vi "Dashboard Cell Resize.vi"(6 "Cluster":T1={"Label Font Size"=24, "Data Font Size"=36, "String Font Size"=36}, 8 "error in (no error)":errorcluster, 9 "Cluster Size:Height":u32=134, 10 "Cluster Size:Width":u32=256, 11 "引气压力P4 4":refnum<vi>) -> (0 "error out":errorcluster, 1 "Bounds:Area Height":u32=134, 2 "Bounds:Area Width":u32=256)   [LabVIEW 2014, in "jkism-tool-support.lvlib"]
uses:
  jkism-tool-support.lvlib
panel:
  out "引气压力P4 2":T2={"Label"="Label", "Value"="0.00", "String"="0.00"} caption="Digital"
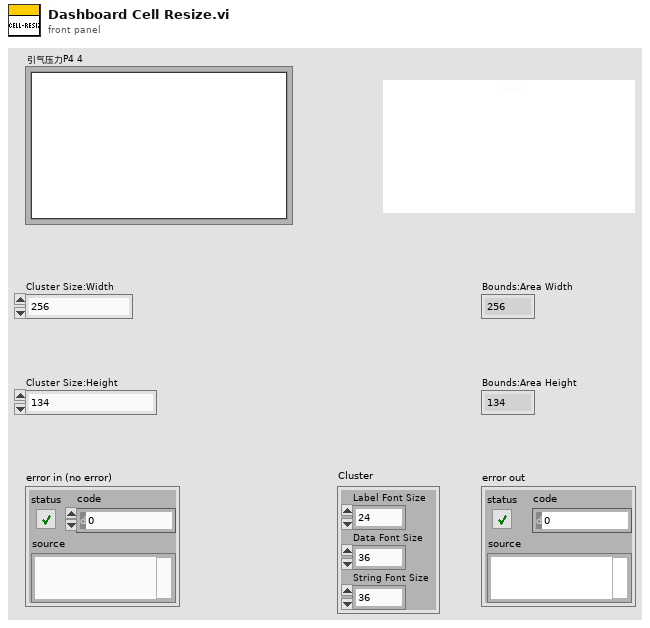
[diagram p1: front panel]
types:
  T1 = cluster{"Label Font Size":i32, "Data Font Size":i32, "String Font Size":i32}
  T2 = cluster{"Label":string, "Value":string, "String":string}
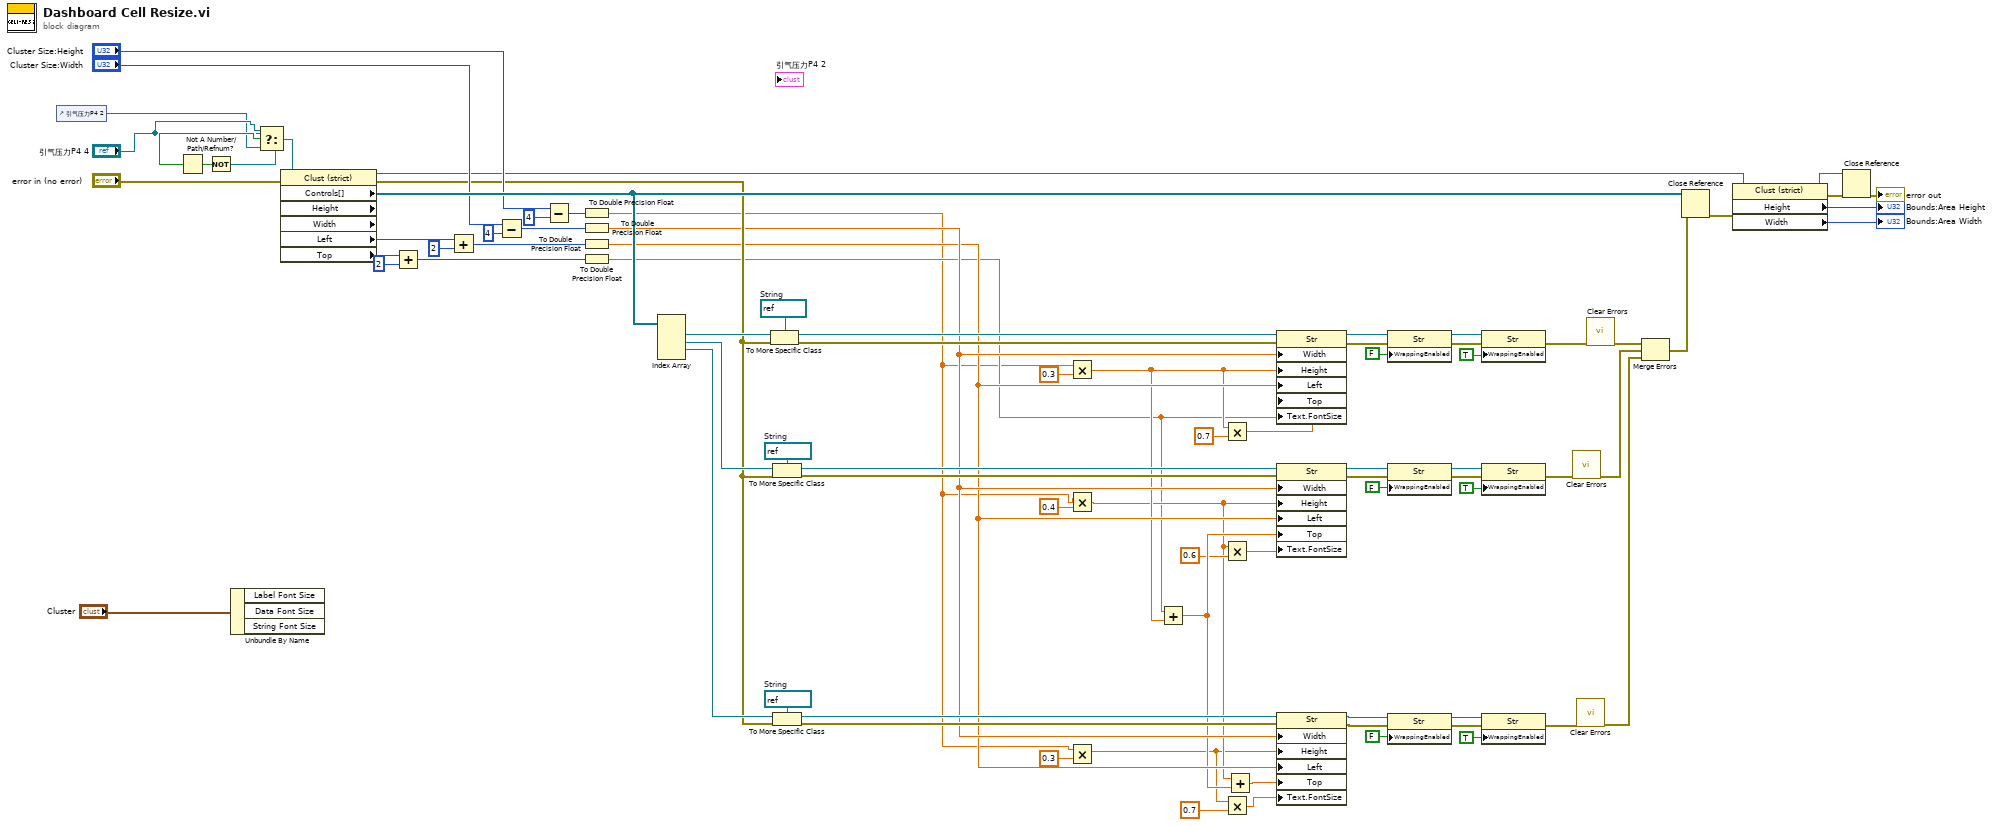
[diagram p0: block diagram]
diagram:
  w47 = refnum<vi> refnum  # String
  w78 = refnum<vi> refnum  # String
  w82 = refnum<vi> refnum  # String
  n1 = control-ref of="引气压力P4 2"() -> (w53:refnum<vi>)
  n2 = Not A Number/Path/Refnum?(number/path/refnum="引气压力P4 4") -> (NaN/Path/Refnum?=w1:bool)
  n3 = Not(x=w1) -> (.not. x?=w55:bool)
  n4 = Unbundle By Name("Cluster") -> ()  [unwired: 3 out]
  n5 = Select(t="引气压力P4 4", s=w55, f=w53) -> (s? t:f=w52:refnum<vi>)
  n6 = property on="Property Node" class="Clust (strict)" props=["Controls[]", "Height", "Width", "Left", "Top"](reference=w52, error in="error in (no error)") -> (reference out=w59:refnum<vi>, error out=w44:errorcluster, "Controls[]"=w83:refnum<vi>[], "Left"=w72:i32, "Top"=w69:i32)  [unwired: 2 out]
  n7 = Add(x=w69, y=2) -> (x+y=w50:i32)
  n8 = Add(x=w72, y=2) -> (x+y=w68:i32)
  n9 = Subtract(x="Cluster Size:Width", y=u32 4) -> (x-y=w75:u32)
  n10 = Subtract(x="Cluster Size:Height", y=u32 4) -> (x-y=w51:u32)
  n11 = To Double Precision Float(number=w51) -> (double precision float=w26:dbl)
  n12 = To Double Precision Float(number=w75) -> (double precision float=w43:dbl)
  n13 = To Double Precision Float(number=w68) -> (double precision float=w42:dbl)
  n14 = To Double Precision Float(number=w50) -> (double precision float=w30:dbl)
  n15 = Index Array(array=w83) -> (element #1=w80:refnum<vi>, element #2=w77:refnum<vi>, element #3=w45:refnum<vi>)  [unwired: 4 in, 1 out]
  n16 = To More Specific Class(target class=w82, reference=w80, error in=w44) -> (specific class reference=w81:refnum<vi>, error out=w65:errorcluster)
  n17 = To More Specific Class(target class=w78, reference=w77, error in=w44) -> (specific class reference=w79:refnum<vi>, error out=w66:errorcluster)
  n18 = To More Specific Class(target class=w47, reference=w45, error in=w44) -> (specific class reference=w46:refnum<vi>, error out=w48:errorcluster)
  n19 = Multiply(x=w26, y=0.3) -> (x*y=w37:dbl)
  n20 = Multiply(x=w26, y=0.4) -> (x*y=w32:dbl)
  n21 = Multiply(x=w26, y=0.3) -> (x*y=w28:dbl)
  n22 = Add(x=w30, y=w37) -> (x+y=w41:dbl)
  n23 = Multiply(x=w37, y=0.7) -> (x*y=w38:dbl)
  n24 = Multiply(x=w32, y=0.6) -> (x*y=w33:dbl)
  n25 = Multiply(x=w28, y=0.7) -> (x*y=w29:dbl)
  n26 = Add(x=w32, y=w41) -> (x+y=w49:dbl)
  n27 = property on="Property Node" class="Str"(reference=w81, error in=w65, "Width"=w43, "Height"=w37, "Left"=w42, "Top"=w30, "Text.FontSize"=w38) -> (reference out=w22:refnum<vi>, error out=w21:errorcluster)
  n28 = property on="Property Node" class="Str"(reference=w79, error in=w66, "Width"=w43, "Height"=w32, "Left"=w42, "Top"=w41, "Text.FontSize"=w33) -> (reference out=w10:refnum<vi>, error out=w11:errorcluster)
  n29 = property on="Property Node" class="Str"(reference=w46, error in=w48, "Width"=w43, "Height"=w28, "Left"=w42, "Top"=w49, "Text.FontSize"=w29) -> (reference out=w4:refnum<vi>, error out=w3:errorcluster)
  n30 = property on="Property Node" class="Str"(reference=w22, error in=w21, "WrappingEnabled"=FALSE ("Enable Wrapping")) -> (reference out=w17:refnum<vi>, error out=w18:errorcluster)
  n31 = property on="Property Node" class="Str"(reference=w10, error in=w11, "WrappingEnabled"=FALSE ("Enable Wrapping")) -> (reference out=w15:refnum<vi>, error out=w14:errorcluster)
  n32 = property on="Property Node" class="Str"(reference=w4, error in=w3, "WrappingEnabled"=FALSE ("Enable Wrapping")) -> (reference out=w5:refnum<vi>, error out=w6:errorcluster)
  n33 = property on="Property Node" class="Str"(reference=w17, error in=w18, "WrappingEnabled"=TRUE ("Enable Wrapping")) -> (error out=w16:errorcluster)  [unwired: 1 out]
  n34 = property on="Property Node" class="Str"(reference=w15, error in=w14, "WrappingEnabled"=TRUE ("Enable Wrapping")) -> (error out=w9:errorcluster)  [unwired: 1 out]
  n35 = property on="Property Node" class="Str"(reference=w5, error in=w6, "WrappingEnabled"=TRUE ("Enable Wrapping")) -> (error out=w2:errorcluster)  [unwired: 1 out]
  n36 = call <vilib>:"Clear Errors.vi"("error in (no error)"=w9) -> ("error out"=w24:errorcluster)  [unwired: 6 in]
  n37 = call <vilib>:"Clear Errors.vi"("error in (no error)"=w2) -> ("error out"=w23:errorcluster)  [unwired: 6 in]
  n38 = call <vilib>:"Clear Errors.vi"("error in (no error)"=w16) -> ("error out"=w25:errorcluster)  [unwired: 6 in]
  n39 = Merge Errors(w25, w24, w23) -> (w76:errorcluster)
  n40 = Close Reference(reference=w83, error in (no error)=w76) -> (error out=w61:errorcluster)
  n41 = property on="Property Node" class="Clust (strict)"(reference=w59, error in=w61) -> (reference out=w58:refnum<vi>, error out=w60:errorcluster, "Height"=→"Bounds:Area Height":u32, "Width"=→"Bounds:Area Width":u32)
  n42 = Close Reference(reference=w58, error in (no error)=w60) -> (error out=→"error out":errorcluster)
